vi "Xml_Save_Expert.vi"(8 "error in (no error)":errorcluster, 11 "Refnum Clust":refnum<vi>) -> (0 "error out":errorcluster, 3 "XML String Out":string[](array[string]))   [LabVIEW 2024]
uses:
  controls/EXPERT_Inputs.ctl
  controls/XML_Inputs.ctl
  controls/SOFTWARE_Inputs.ctl
  controls/HSDIO_6541_Inputs.ctl
  <instrlib>/niHSDIO/niHSDIO.llb/niHSDIO_ctl Trigger Source Values (Ring).ctl
  controls/AWG_5421_Inputs.ctl
  <instrlib>/niFgen/niFgen.llb/niFgen_ctl Trigger Source Values (Ring).ctl
  controls/DIGIT_5122_Inputs.ctl
  <instrlib>/niScope/Controls/niScope trigger source.ctl
  controls/AO_6711_Inputs.ctl
  controls/AO_6738_Inputs.ctl
  controls/HARDWARE_Inputs.ctl
panel:
  in  "HARDWARE Inputs":T1={"AO 6711 Inputs"={"Physical Channels"="AO_6711/ao0:3", "Min Voltage"=-10.0, "Max Voltage"=10.0, "Trigger Source"="/AO_6711/PFI3", "Counter"="AO_6711/ctr0"}, "AO 6738 Inputs"={"Physical Channels"="AO_6738/ao0:3", "Min Voltage"=-10.0, "Max Voltage"=10.0, "Trigger Source"="/AO_6738/PFI2", "Counter"="AO_6738/ctr0"}, "AWG 5421 Inputs"={"Resource Name"="AWG_5421", "Sample Rate"=10000000.0, "Trigger Type"=2, "Trigger Source"="PFI0", "Waveform Gain"=0.31, "Digital Filter ON"=TRUE}, "DIGIT 5122 Inputs"={"Sample Rate"=10000.0, "Resource Name"="DIGIT_5122", "Channel Name"="0", "Trigger Source"="VAL_EXTERNAL", "Vertical Range"=10.0, "Trigger Level"=3.0}, "HSDIO 6541 Inputs"={"Resource Name"="HSDIO_6541", "Clock Rate"=1000000.0, "Trigger Source"="PFI0"}} {"AO 6738 Inputs"."Max Voltage" min=-10.0 max=10.0; "AO 6738 Inputs"."Min Voltage" min=-10.0 max=10.0; "HSDIO 6541 Inputs"."Clock Rate" format="%.2p"; "DIGIT 5122 Inputs"."Trigger Level" format="%.2f"; "DIGIT 5122 Inputs"."Vertical Range" format="%.2f"; "DIGIT 5122 Inputs"."Sample Rate" step=65535.0 format="%#_3p"; "AWG 5421 Inputs"."Sample Rate" format="%.2p"; "AWG 5421 Inputs"."Trigger Type" items=["None", "Software Edge", "Digital Edge", "Digital Level"]; "AO 6711 Inputs"."Max Voltage" min=-10.0 max=10.0; "AO 6711 Inputs"."Min Voltage" min=-10.0 max=10.0}
  in  "EXPERT Inputs":T10={"XML Inputs"={"Version Tag Name"="XML_Version", "Version String"="1.0"}, "SOFTWARE Inputs"={"Application Directory"=path "D:/S.O.F.T.S/LABVIEW/PIL", "Software Version"="1.0.0", "Data Path"=path "D:/PIRENEA/DATA", "XML Path"=path "D:/PIRENEA/DATA", "XML File Filter"="*.xml", "XML Saved Path"=path "D:/PIRENEA/DATA/SAVED", "Excit Scripts Path"=path "D:/PIRENEA/EXCIT_SCRIPTS", "Excit Scripts File Filter"="*.txt", "Excit Waveforms Path"=path "D:/PIRENEA/EXCIT_WFMS", "Excit Waveforms File Filter"="*.bin", "Timing Scripts Path"=path "D:/PIRENEA/TIMING_SCRIPTS", "Timing Scripts File Filter"="*.txt", "Timing Waveforms Path"=path "D:/PIRENEA/TIMING_WFMS", "Timing Waveforms File Filter"="*.bin", "Trapping Waveforms Path"=path "D:/PIRENEA/TRAPPING_WFMS", "Trapping Waveforms File Filter"="*.bin"}, "HSDIO 6541 Inputs"={"Resource Name"="HSDIO_6541", "Clock Rate"=1000000.0, "Trigger Source"="PFI0"}, "AWG 5421 Inputs"={"Resource Name"="AWG_5421", "Sample Rate"=10000000.0, "Trigger Type"=2, "Trigger Source"="PFI0", "Waveform Gain"=0.31, "Digital Filter ON"=TRUE}, "DIGIT 5122 Inputs"={"Sample Rate"=10000.0, "Resource Name"="DIGIT_5122", "Channel Name"="0", "Trigger Source"="VAL_EXTERNAL", "Vertical Range"=10.0, "Trigger Level"=3.0}, "AO 6711 Inputs"={"Physical Channels"="AO_6711/ao0:3", "Min Voltage"=-10.0, "Max Voltage"=10.0, "Trigger Source"="/AO_6711/PFI3", "Counter"="AO_6711/ctr0"}, "AO 6738 Inputs"={"Physical Channels"="AO_6738/ao0:3", "Min Voltage"=-10.0, "Max Voltage"=10.0, "Trigger Source"="/AO_6738/PFI2", "Counter"="AO_6738/ctr0"}} {"AO 6738 Inputs"."Max Voltage" min=-10.0 max=10.0; "AO 6738 Inputs"."Min Voltage" min=-10.0 max=10.0; "AWG 5421 Inputs"."Sample Rate" format="%.2p"; "AWG 5421 Inputs"."Trigger Type" items=["None", "Software Edge", "Digital Edge", "Digital Level"]; "AO 6711 Inputs"."Max Voltage" min=-10.0 max=10.0; "AO 6711 Inputs"."Min Voltage" min=-10.0 max=10.0; "HSDIO 6541 Inputs"."Clock Rate" format="%.2p"; "DIGIT 5122 Inputs"."Trigger Level" format="%.2f"; "DIGIT 5122 Inputs"."Vertical Range" format="%.2f"; "DIGIT 5122 Inputs"."Sample Rate" step=65535.0 format="%#_3p"}
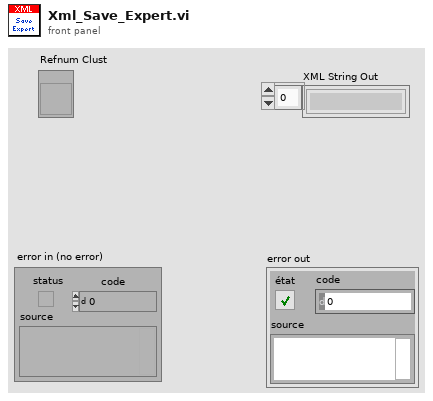
[diagram p1: front panel]
types:
  T1 = typedef "HARDWARE_Inputs.ctl" = cluster{"AO 6711 Inputs":T2, "AO 6738 Inputs":T3, "AWG 5421 Inputs":T4, "DIGIT 5122 Inputs":T6, "HSDIO 6541 Inputs":T8}
  T2 = typedef "AO_6711_Inputs.ctl" = cluster{"Physical Channels":tag, "Min Voltage":dbl, "Max Voltage":dbl, "Trigger Source":tag, "Counter":tag}
  T3 = typedef "AO_6738_Inputs.ctl" = cluster{"Physical Channels":tag, "Min Voltage":dbl, "Max Voltage":dbl, "Trigger Source":tag, "Counter":tag}
  T4 = typedef "AWG_5421_Inputs.ctl" = cluster{"Resource Name":refnum<k15>, "Sample Rate":dbl, "Trigger Type":u16, "Trigger Source":T5, "Waveform Gain":dbl, "Digital Filter ON":bool}
  T5 = typedef "niFgen_ctl Trigger Source Values (Ring).ctl" = string
  T6 = typedef "DIGIT_5122_Inputs.ctl" = cluster{"Sample Rate":dbl, "Resource Name":refnum<k15>, "Channel Name":string, "Trigger Source":T7, "Vertical Range":dbl, "Trigger Level":dbl}
  T7 = typedef "niScope trigger source.ctl" = string
  T8 = typedef "HSDIO_6541_Inputs.ctl" = cluster{"Resource Name":refnum<k15>, "Clock Rate":dbl, "Trigger Source":T9}
  T9 = typedef "niHSDIO_ctl Trigger Source Values (Ring).ctl" = string
  T10 = typedef "EXPERT_Inputs.ctl" = cluster{"XML Inputs":T11, "SOFTWARE Inputs":T12, "HSDIO 6541 Inputs":T8, "AWG 5421 Inputs":T4, "DIGIT 5122 Inputs":T6, "AO 6711 Inputs":T2, "AO 6738 Inputs":T3}
  T11 = typedef "XML_Inputs.ctl" = cluster{"Version Tag Name":string, "Version String":string}
  T12 = typedef "SOFTWARE_Inputs.ctl" = cluster{"Application Directory":path, "Software Version":string, "Data Path":path, "XML Path":path, "XML File Filter":string, "XML Saved Path":path, "Excit Scripts Path":path, "Excit Scripts File Filter":string, "Excit Waveforms Path":path, "Excit Waveforms File Filter":string, "Timing Scripts Path":path, "Timing Scripts File Filter":string, "Timing Waveforms Path":path, "Timing Waveforms File Filter":string, "Trapping Waveforms Path":path, "Trapping Waveforms File Filter":string}
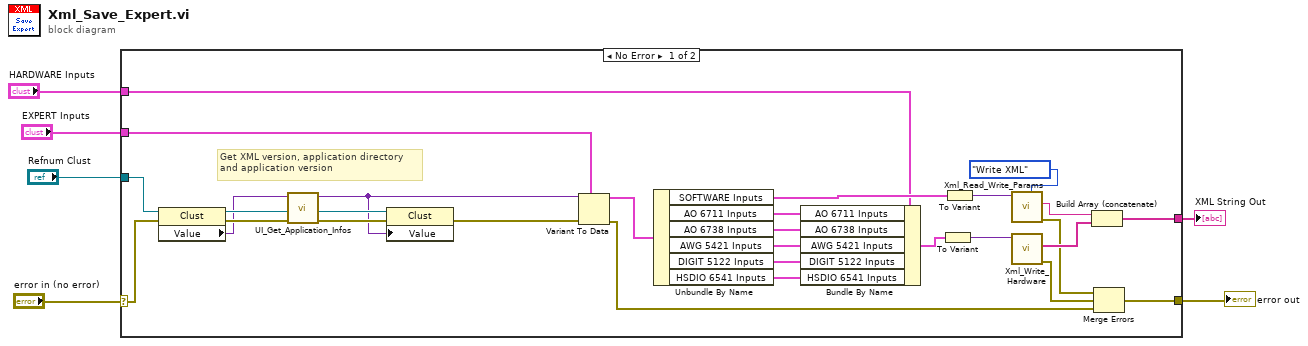
[diagram p0: block diagram]
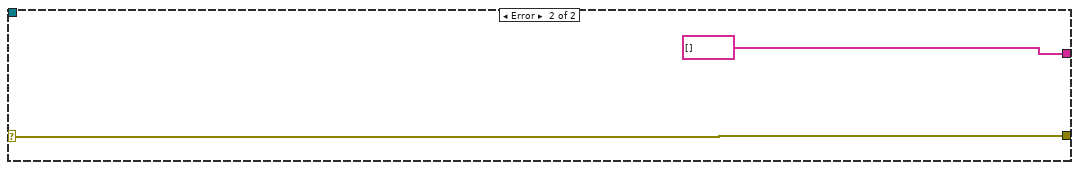
[diagram p2: hidden frame]
diagram:
  n1 = case shown="No Error" "error in (no error)" {
    selector: "error in (no error)" -> [w12 w36]
    tunnel: [w34 w36] -> w5
    tunnel: [w33 string[] []] -> w3
    tunnel: "Refnum Clust" -> [w17 _]
    tunnel: "EXPERT Inputs" -> [w16 _]
    tunnel: "HARDWARE Inputs" -> [w15 _]
    frame No Error {
      # "Get XML version, application directory\nand application version"
      n2 = property class="Clust"(reference=w17, error in=w12) -> (reference out=w13:refnum<vi>, error out=w11:errorcluster, "Value"=w10:variant)
      n3 = call "UI_Get_Application_Infos.vi"("error in (no error)"=w11, "Variant"=w10) -> ("error out"=w14:errorcluster, "Variant Output"=w9:variant)  [unwired: 8 in]
      n4 = property class="Clust"(reference=w13, error in=w14, "Value"=w9) -> (error out=w8:errorcluster)  [unwired: 1 out]
      n5 = Variant To Data(error in=w8, type=w16, Variant=w9) -> (data=w27:T10, error out=w20:errorcluster)
      n6 = Unbundle By Name(w27) -> ("SOFTWARE Inputs"=w29:T12, "AO 6711 Inputs"=w26:T2, "AO 6738 Inputs"=w25:T3, "AWG 5421 Inputs"=w24:T4, "DIGIT 5122 Inputs"=w23:T6, "HSDIO 6541 Inputs"=w7:T8)
      n7 = Bundle By Name(cluster=w15, "AO 6711 Inputs"=w26, "AO 6738 Inputs"=w25, "AWG 5421 Inputs"=w24, "DIGIT 5122 Inputs"=w23, "HSDIO 6541 Inputs"=w7) -> (w22:T1)
      n8 = To Variant(anything=w22) -> (Variant=w30:variant)
      n9 = To Variant(anything=w29) -> (Variant=w32:variant)
      n10 = call "Xml_Read_Write_Params.vi"("Variant"=w32, "Command"=enum16{"Read XML", "Set", "Get", "Write XML"}."Write XML") -> ("XML String Out"=w28:string, "error out"=w18:errorcluster)  [unwired: 5 in, 1 out]
      n11 = call "Xml_Write_Hardware.vi"("Variant"=w30) -> ("error out"=w19:errorcluster, "XML String Out"=w21:string[])  [unwired: 8 in, 1 out]
      n12 = Build Array (concatenate)(w28, w21) -> (w33:string[])
      n13 = Merge Errors(w18, w19, w20) -> (w34:errorcluster)
    }
    frame Error {
    }
  }
  "error out" <- w5
  "XML String Out" <- w3
